vi "링컨트롤.vi"() -> ()   [LabVIEW 2014]
panel:
  out "초 단위":dbl
  in  "시간입력":dbl
  in  "링":u32(ring) items=["일"=86400, "시간"=3600, "분"=60, "초"=1]
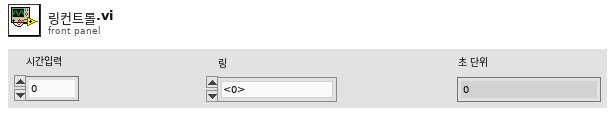
[diagram p1: front panel]
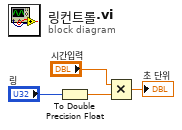
[diagram p0: block diagram]
diagram:
  n1 = To Double Precision Float(number="링") -> (double precision float=w2:dbl)
  n2 = Multiply(x="시간입력", y=w2) -> (x*y=→"초 단위":dbl)
